vi "Read System Configuration.vi"(8 "error in (no error)":errorcluster, 11 "System Configuration File Path":path) -> (0 "error out":errorcluster, 3 "System Configuration":T1)   [LabVIEW 2024]
doc: "Reads the system configuration from the configuration file."
uses:
  Controls/Server/System Configuration.ctl
  Controls/Server/Subsystem Configuration.ctl
  <vilib>/Utility/config.llb/Read Key (String).vi
  <vilib>/Utility/config.llb/Read Key (Path).vi
  <vilib>/Utility/config.llb/Read Key (Boolean).vi
  <vilib>/Utility/config.llb/Read Key (U32).vi
  <vilib>/Utility/config.llb/NI_LVConfig.lvlib
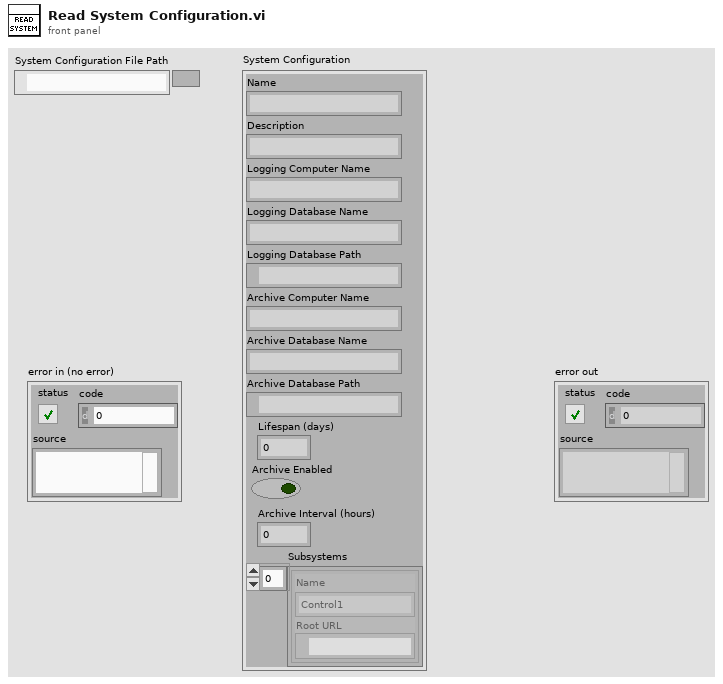
[diagram p1: front panel]
types:
  T1 = typedef "System Configuration.ctl" = cluster{"Name":string, "Description":string, "Logging Computer Name":string, "Logging Database Name":string, "Logging Database Path":path, "Archive Computer Name":string, "Archive Database Name":string, "Archive Database Path":path, "Lifespan (days)":u32, "Archive Enabled":bool, "Archive Interval (hours)":u32, "Subsystems":T2[]}
  T2 = typedef "Subsystem Configuration.ctl" = cluster{"Name":string, "Root URL":refnum<k21>}
  T3 = typedef "NI_LVConfig.lvlib/Config Data RefNum.ctl" = refnum<k1>
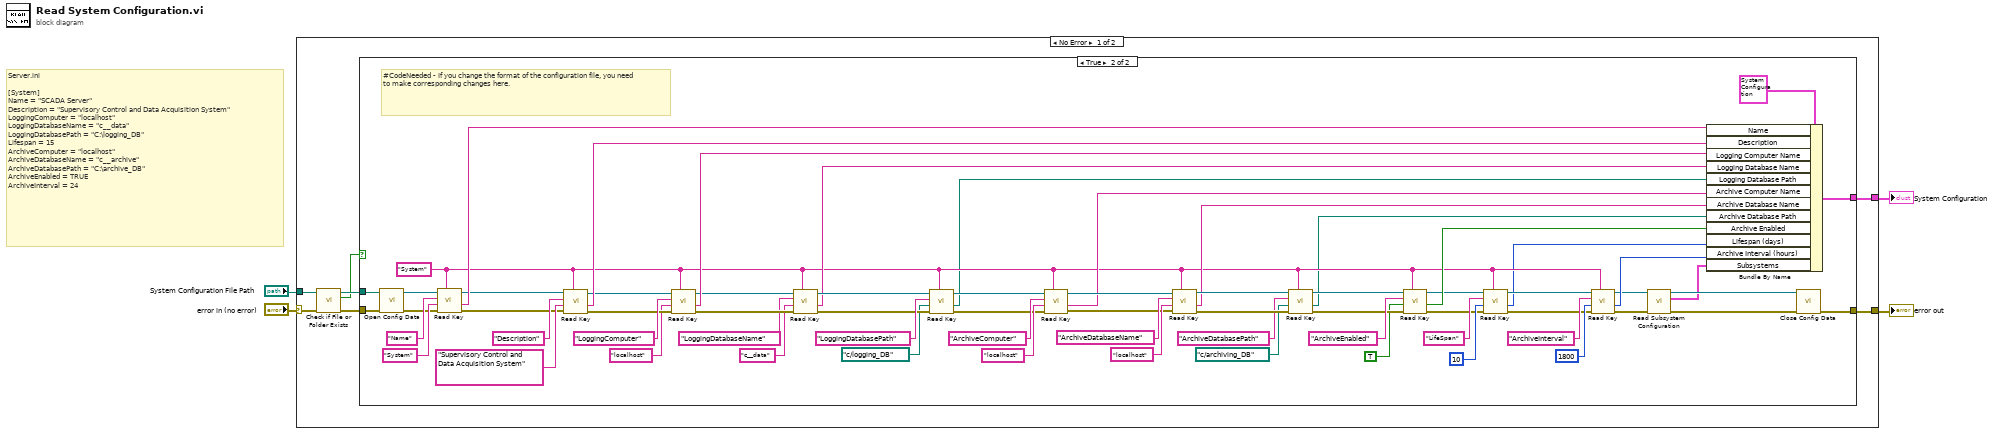
[diagram p0: block diagram]
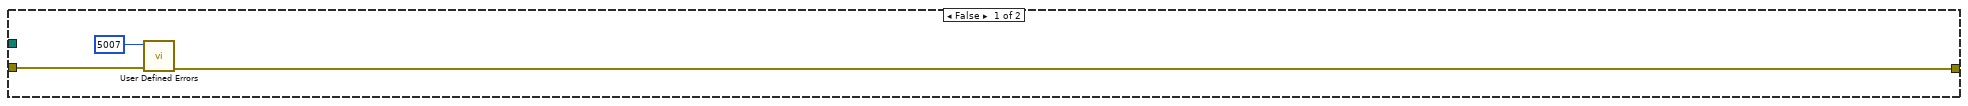
[diagram p2: hidden frame]
diagram:
  # "Server.ini\n\n[System]\nName = \"SCADA Server\"\nDescription = \"Supervisory Control and Data Acquisition System\"\nLoggingComputer = \"localhost\"\nLoggingDatabaseName = \"c__data\"\nLoggingDatabasePath = \"C:\\logging_DB\"\nLifespan = 15    \nArchiveComputer = \"localhost\"\nArchiveDatabaseName = \"c__archive\"\nArchiveDatabasePath = \"C:\\archive_DB\"\nArchiveEnabled = TRUE    \nArchiveInterval = 24"
  n1 = case shown="No Error" "error in (no error)" {
    selector: "error in (no error)" -> [w7 w81]
    tunnel: [w11 w81] -> w4
    tunnel: [w10 _] -> w3
    tunnel: "System Configuration File Path" -> [w8 _]
    frame No Error {
      n2 = call <vilib>:"Check if File or Folder Exists.vi"("error in (no error)"=w7, "path"=w8) -> ("error out"=w6:errorcluster, "file or folder exists?"=w5:bool, "dup path"=w9:path)  [unwired: 7 in]
      n3 = case shown="True" w5 {
        tunnel: w6 -> [w12 w19]
        tunnel: [w13 w78] -> w11
        tunnel: [_ w24] -> w10
        tunnel: w9 -> [_ w20]
        frame False {
          n4 = call "User Defined Errors.vi"("error in (no error)"=w12, "Error Code (0)"=5007 ("error code (0)")) -> ("error out"=w13:errorcluster)  [unwired: 9 in]
        }
        frame True {
          w30 = "System" ("section")
          # "#CodeNeeded - If you change the format of the configuration file, you need to make corresponding changes here."
          n5 = call <vilib>:"Open Config Data.vi"("error in (no error)"=w19, "configuration file path"=w20) -> ("error out"=w21:errorcluster, "refnum"=w22:T3)  [unwired: 7 in, 1 out]
          n6 = call-poly <vilib>:"Read Key.vi"("section"=w30, "error in (no error)"=w21, "default value"="System", "key"="Name", "refnum"=w22) -> ("error out"=w71:errorcluster, "value"=w75:string, "refnum out"=w72:T3)  [unwired: 3 in, 1 out]
          n7 = call-poly <vilib>:"Read Key.vi"("section"=w30, "error in (no error)"=w71, "default value"="Supervisory Control and Data Acquisition System", "key"="Description", "refnum"=w72) -> ("error out"=w67:errorcluster, "value"=w70:string, "refnum out"=w68:T3)  [unwired: 3 in, 1 out]
          n8 = call-poly <vilib>:"Read Key.vi"("section"=w30, "error in (no error)"=w67, "default value"="localhost", "key"="LoggingComputer", "refnum"=w68) -> ("error out"=w50:errorcluster, "value"=w65:string, "refnum out"=w48:T3)  [unwired: 3 in, 1 out]
          n9 = call-poly <vilib>:"Read Key.vi"("section"=w30, "error in (no error)"=w50, "default value"="c__data", "key"="LoggingDatabaseName", "refnum"=w48) -> ("error out"=w49:errorcluster, "value"=w46:string, "refnum out"=w47:T3)  [unwired: 3 in, 1 out]
          n10 = call-poly <vilib>:"Read Key.vi"("section"=w30, "error in (no error)"=w49, "default value"=path "c:/logging_DB", "key"="LoggingDatabasePath", "refnum"=w47) -> ("error out"=w41:errorcluster, "value"=w18:path, "refnum out"=w39:T3)  [unwired: 3 in, 1 out]
          n11 = call-poly <vilib>:"Read Key.vi"("section"=w30, "error in (no error)"=w41, "default value"="localhost", "key"="ArchiveComputer", "refnum"=w39) -> ("error out"=w40:errorcluster, "value"=w37:string, "refnum out"=w38:T3)  [unwired: 3 in, 1 out]
          n12 = call-poly <vilib>:"Read Key.vi"("section"=w30, "error in (no error)"=w40, "default value"="localhost", "key"="ArchiveDatabaseName", "refnum"=w38) -> ("error out"=w63:errorcluster, "value"=w58:string, "refnum out"=w62:T3)  [unwired: 3 in, 1 out]
          n13 = call-poly <vilib>:"Read Key.vi"("section"=w30, "error in (no error)"=w63, "default value"=path "c:/archiving_DB", "key"="ArchiveDatabasePath", "refnum"=w62) -> ("error out"=w53:errorcluster, "value"=w15:path, "refnum out"=w54:T3)  [unwired: 3 in, 1 out]
          n14 = call-poly <vilib>:"Read Key.vi"("section"=w30, "error in (no error)"=w53, "default value"=TRUE, "key"="ArchiveEnabled", "refnum"=w54) -> ("error out"=w33:errorcluster, "value"=w51:bool, "refnum out"=w34:T3)  [unwired: 3 in, 1 out]
          n15 = call-poly <vilib>:"Read Key.vi"("section"=w30, "error in (no error)"=w33, "default value"=u32 10, "key"="LifeSpan", "refnum"=w34) -> ("error out"=w32:errorcluster, "value"=w29:u32, "refnum out"=w31:T3)  [unwired: 3 in, 1 out]
          n16 = call-poly <vilib>:"Read Key.vi"("section"=w30, "error in (no error)"=w32, "default value"=u32 1800, "key"="ArchiveInterval", "refnum"=w31) -> ("error out"=w26:errorcluster, "value"=w28:u32, "refnum out"=w23:T3)  [unwired: 3 in, 1 out]
          n17 = call "Read Subsystem Configuration.vi"("error in (no error)"=w26, "Configuration Refnum In"=w23) -> ("error out"=w79:errorcluster, "Subsystems"=w25:T2[], "Configuration Refnum Out"=w80:T3)  [unwired: 7 in]
          n18 = Bundle By Name(cluster=T1 {"Name"="", "Description"="", "Logging Computer Name"="", "Logging Database Name"="", "Logging Database Path"=path "", "Archive Computer Name"="", "Archive Database Name"="", "Archive Database Path"=path "", "Lifespan (days)"=0, "Archive Enabled"=FALSE, "Archive Interval (hours)"=0, "Subsystems"=[]} ("Cluster"), "Name"=w75, "Description"=w70, "Logging Computer Name"=w65, "Logging Database Name"=w46, "Logging Database Path"=w18, "Archive Computer Name"=w37, "Archive Database Name"=w58, "Archive Database Path"=w15, "Archive Enabled"=w51, "Lifespan (days)"=w29, "Archive Interval (hours)"=w28, "Subsystems"=w25) -> (w24:T1)
          n19 = call <vilib>:"Close Config Data.vi"("error in (no error)"=w79, "refnum"=w80) -> ("error out"=w78:errorcluster)  [unwired: 8 in, 1 out]
        }
      }
    }
    frame Error {
    }
  }
  "error out" <- w4
  "System Configuration" <- w3
